vi "permissions_set-attrib.vi"(6 "recursive?":bool, 8 "error in (no error)":errorcluster, 9 "attributes_to_remove []":T1[](array[typedef]), 10 "attributes_to_add []":T1[](array[typedef]), 11 "filepath in":path) -> (0 "error out":errorcluster, 3 "filepath out":path)   [LabVIEW 2015, in "lv-bin-windows.lvlib" / "v1.lvlib"]
uses:
  v1.lvlib
  _controls/attribute.ctl
  <userlib>/antonio-alexander/lv-bin/lv-bin/public/api/v1/v1.lvlib
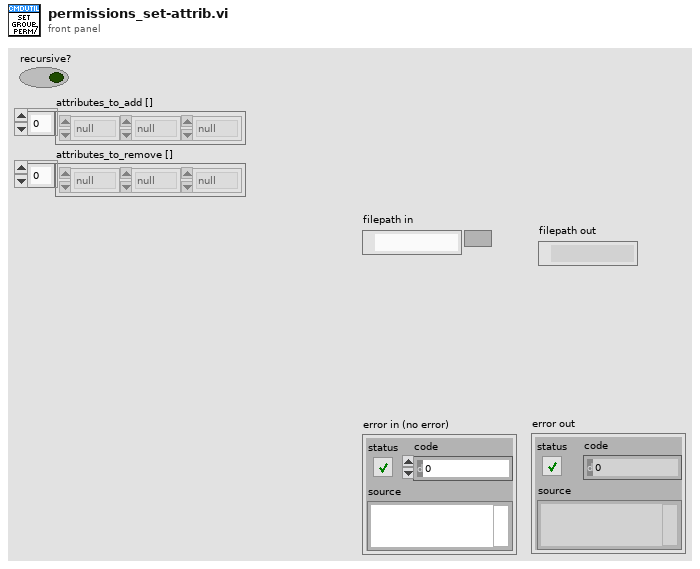
[diagram p1: front panel]
types:
  T1 = typedef "lv-bin-windows.lvlib/v1.lvlib/attribute.ctl" = enum16{"null", "read", "archive", "system", "hidden", "index"}
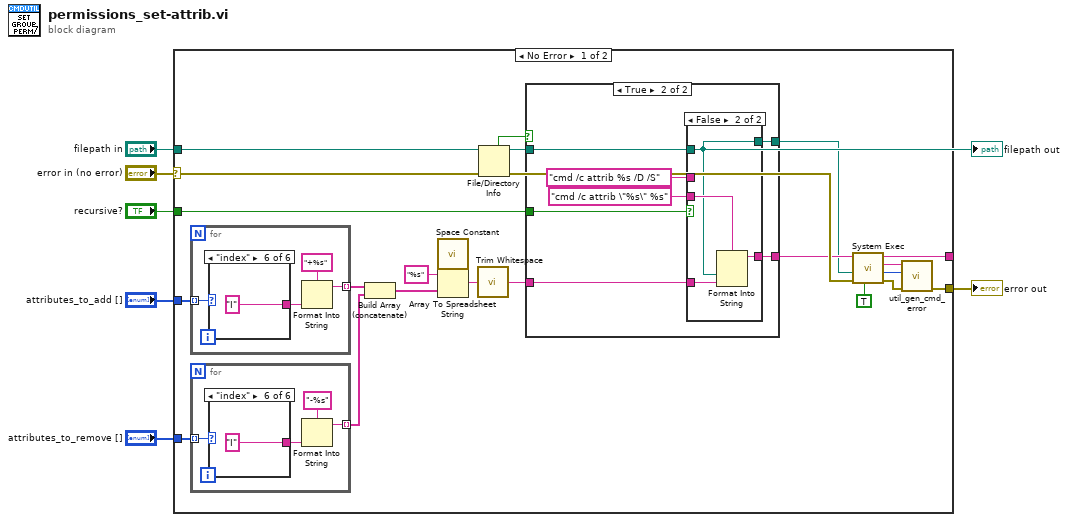
[diagram p0: block diagram]
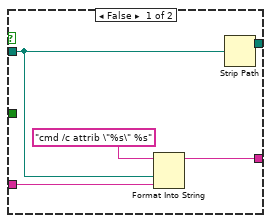
[diagram p2: hidden frame]
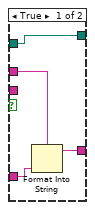
[diagram p3: hidden frame]
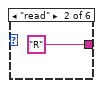
[diagram p5: hidden frame]
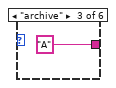
[diagram p6: hidden frame]
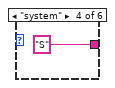
[diagram p7: hidden frame]
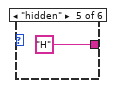
[diagram p8: hidden frame]
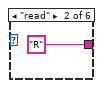
[diagram p10: hidden frame]
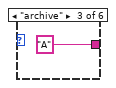
[diagram p11: hidden frame]
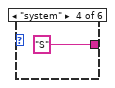
[diagram p12: hidden frame]
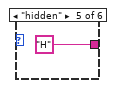
[diagram p13: hidden frame]
diagram:
  n1 = case shown="No Error" "error in (no error)" {
    selector: "error in (no error)" -> [w13 w67]
    tunnel: [w29 w67] -> w6
    tunnel: "filepath in" -> [w14 _]
    tunnel: "attributes_to_add []" -> [w24 _]
    tunnel: "attributes_to_remove []" -> [w23 _]
    tunnel: "recursive?" -> [w16 _]
    tunnel: [w15 _] -> _
    frame No Error {
      n2 = for {
        tunnel: w24 -> [w61] mode=indexing
        tunnel: [w58] -> w22 mode=indexing
        n3 = case shown="\"index\"" w61 {
          tunnel: [_ "R" "A" "S" "H" "I"] -> w60
          frame Default {
          }
          frame "read" {
          }
          frame "archive" {
          }
          frame "system" {
          }
          frame "hidden" {
          }
          frame "index" {
          }
        }
        n4 = Format Into String(format string="+%s", w60) -> (resulting string=w58:string)  [unwired: 2 in, 1 out]
      }
      n5 = for {
        tunnel: w23 -> [w52] mode=indexing
        tunnel: [w49] -> w21 mode=indexing
        n6 = case shown="\"index\"" w52 {
          tunnel: [_ "R" "A" "S" "H" "I"] -> w51
          frame Default {
          }
          frame "read" {
          }
          frame "archive" {
          }
          frame "system" {
          }
          frame "hidden" {
          }
          frame "index" {
          }
        }
        n7 = Format Into String(format string="-%s", w51) -> (resulting string=w49:string)  [unwired: 2 in, 1 out]
      }
      n8 = Build Array (concatenate)(w22, w21) -> (w20:string[])
      n9 = call <vilib>:"Space Constant.vi"() -> ("String"=w18:string)
      n10 = Array To Spreadsheet String(delimiter (Tab)=w18, array=w20, 3:"%s" ("format string")) -> (spreadsheet string=w17:string)
      n11 = call <vilib>:"Trim Whitespace.vi"("string"=w17) -> ("trimmed string"=w10:string)  [unwired: 1 in]
      n12 = File/Directory Info(path=w14, error in=w13) -> (path out=w9:path, directory=w12:bool, error out=w11:errorcluster)  [unwired: 4 out]
      n13 = case shown="True" w12 {
        tunnel: [w33 w40] -> w8
        tunnel: w16 -> [_ w39]
        tunnel: w10 -> [w32 w35]
        tunnel: w9 -> [w31 w36]
        tunnel: [w30 w34] -> w7
        frame False {
          w33 = "cmd /c attrib \"%s\" %s"
          n14 = Format Into String(format string=w33, w31, w32) -> ()  [unwired: 2 in, 2 out]
          n15 = Strip Path(path=w31) -> (stripped path=w30:path)  [unwired: 1 out]
        }
        frame True {
          n16 = case shown="False" w39 {
            tunnel: [w44 w48] -> w40
            tunnel: "cmd /c attrib \"%s\" %s" -> [_ w47]
            tunnel: "cmd /c attrib %s /D /S" -> [w43 _]
            tunnel: w36 -> [w41 w45]
            tunnel: w35 -> [w42 w46]
            tunnel: [w41 w45] -> w34
            frame True {
              n17 = Format Into String(format string=w43, w42) -> (resulting string=w44:string)  [unwired: 2 in, 1 out]
            }
            frame False {
              n18 = Format Into String(format string=w47, w45, w46) -> (resulting string=w48:string)  [unwired: 2 in, 1 out]
            }
          }
        }
      }
      n19 = call <vilib>:"System Exec.vi"("run minimized? (F)"=TRUE, "error in (no error)"=w11, "working directory"=w7, "command line"=w8) -> ("error out"=w27:errorcluster, "return code"=w25:i32, "standard error"=w26:string, "standard output"=w15:string)  [unwired: 4 in]
      n20 = call <userlib>:"util_gen_cmd_error.vi"("error in (no error)"=w27, "return_code"=w25, "standard_error"=w26) -> ("error out"=w29:errorcluster)  [unwired: 8 in]
    }
    frame Error {
    }
  }
  "error out" <- w6
  "filepath out" <- "filepath in"
